vi "Config Core.vi"(8 "Error In":errorcluster, 10 "IConfig In":refnum<class "IConfig.lvclass">, 11 "Hardware In":refnum<class "IRef.lvclass">) -> (0 "Error Out":errorcluster, 2 "IConfig Out":refnum<class "IConfig.lvclass">, 3 "Hardware Out":refnum<class "IRef.lvclass">)   [LabVIEW 2020, in "IConfig.lvclass"]
uses:
  IConfig.lvclass
  IReference/IRef.lvclass
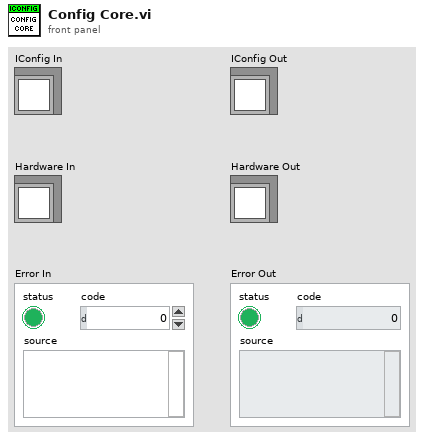
[diagram p1: front panel]
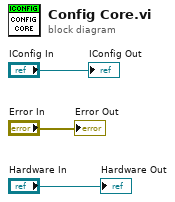
[diagram p0: block diagram]
diagram:
  "Error Out" <- "Error In"
  "Hardware Out" <- "Hardware In"
  "IConfig Out" <- "IConfig In"
